vi "4 Analog Out.vi"() -> ()   [LabVIEW 2015]
uses:
  <vilib>/LabVIEW Interface for Arduino/Type Defs/Board Type.ctl
  <vilib>/LabVIEW Interface for Arduino/Type Defs/Connection Type.ctl
  <vilib>/LabVIEW Interface for Arduino/LabVIEW Interface for Arduino.lvlib
panel:
  in  "VISA resource":refnum<visa-resource-name>="COM10"
  in  "Pin No":u8=3
  in  "Duty Cycle (0 - 255)":u8(knob) scale=0.0..255.0
  in  "Stop":bool
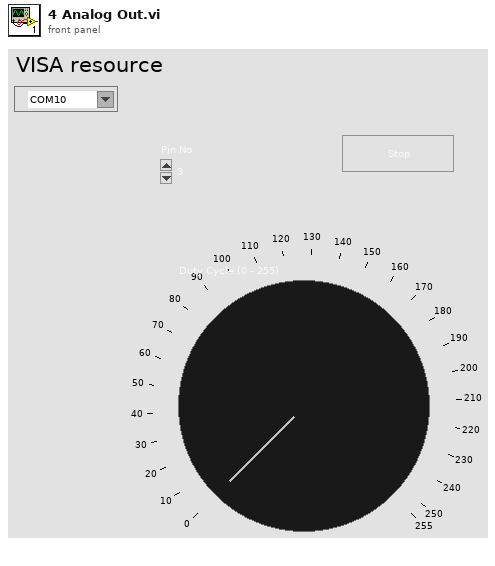
[diagram p1: front panel]
types:
  T1 = typedef "LabVIEW Interface for Arduino.lvlib/Connection Type.ctl" = enum8{"USB / Serial", "XBEE", "BlueSmirf (Bluetooth)"}
  T2 = typedef "LabVIEW Interface for Arduino.lvlib/Board Type.ctl" = enum16{"Uno", "Dimuelanove w/Atmega 328", "Mega 2560"}
  T3 = typedef "LabVIEW Interface for Arduino.lvlib/Arduino Resource.ctl" = cluster{"VISA resource":refnum<visa-resource-name>, "Board Type":T2, "Connection Type":enum8{"USB / Serial"}, "Bytes Per Packet (15)":u8}
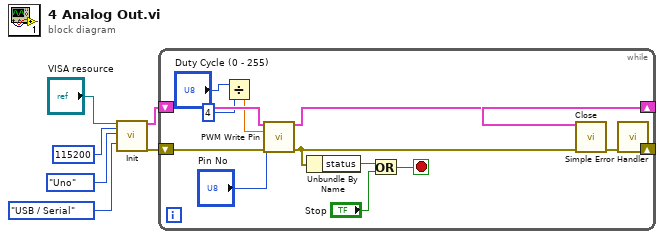
[diagram p0: block diagram]
diagram:
  n1 = call <vilib>:"Init.vi"("VISA resource"="VISA resource", "Baud Rate (115200)"=u32 115200, "Board Type (Uno)"=Board_Type."Uno", "Connection Type (USB/Serial)"=Connection_Type."USB / Serial") -> ("Arduino Resource"=w9:T3, "error out"=w6:errorcluster)  [unwired: 14 in]
  n2 = while {
    shift-right: [w20] -> w8
    shift-left: w9 -> [w16]
    shift-right: [w19] -> w7
    shift-left: w6 -> [w15]
    stop <- w14 stop-if-true
    n3 = Divide(x="Duty Cycle (0 - 255)", y=u8 4) -> (x/y=w10:dbl)
    n4 = call <vilib>:"PWM Write Pin.vi"("Arduino Resource"=w16, "Duty Cycle (0 - 255)"=w10, "PWM Pin (3)"="Pin No", "error in"=w15) -> ("Arduino Resource"=w20:T3, "error out"=w19:errorcluster)  [unwired: 10 in]
    n5 = Unbundle By Name(w19) -> ("status"=w18:bool)
    n6 = Or(x=w18, y="Stop") -> (x .or. y?=w14:bool)
  }
  n7 = call <vilib>:"Close.vi"("Arduino Resource"=w8, "error in"=w7) -> ("error out"=w5:errorcluster)  [unwired: 13 in]
  n8 = call <vilib>:"Simple Error Handler.vi"("error in (no error)"=w5) -> ()  [unwired: 4 in, 5 out]
